vi "vipm_build.vi"   [LabVIEW 2020]
uses:
  <vilib>/Comparison/Equal/Equal Functor/Equal Functor.lvclass
  <vilib>/regexp/Match Regular Expression.xnode
  <vilib>/Wiresmith Technology/G CLI/CLI Class/CLI.lvclass
  <vilib>/Wiresmith Technology/G CLI/Argument Parser/Option Set Class/Option Set.lvclass
  <vilib>/Wiresmith Technology/G CLI/Argument Parser/Option Class/Argument Type.ctl
  <vilib>/Wiresmith Technology/G CLI/Argument Parser/Option Class/Option.lvclass
  <vilib>/Wiresmith Technology/G CLI/Argument Parser/Option Class/Option Configuration.ctl
  094f6021-4ef8-4573-82ce-a7b4949f6c5c.vi
  6795289f-0a04-455c-a499-a5e59a361415.vi
  <vilib>/Utility/error.llb/DialogType.ctl
  35111923-3b9e-4c36-b72b-79289da6bcaf.vi
  0b828e9d-cbba-40c4-b017-a79c080be190.vi
  <resource>/dialog/lvconfig.llb/LV Config Write String.vi
  <resource>/dialog/lvconfig.llb/LV Config Write Numeric (I32).vi
  <resource>/dialog/lvconfig.llb/LV Config Write Color.vi
  <resource>/dialog/lvconfig.llb/LV Config Write Pathlist.vi
  <vilib>/JKI/VIPM API/VIPM API_vipm_api.lvlib
  <resource>/dialog/lvconfig.llb/LV Config Write Boolean.vi
  0a0c95df-62a9-4167-843d-69168cea43e8.vi
  611b17c5-4e93-4ed1-8d2f-f8190cd7dade.vi
types:
  T1 = cluster{"VerboseMode":bool, "Operation":string, "Arguments":string[], "VipbFile":path}
  T2 = enum32{"Invalid", "Standard", "Closed", "Hidden", "Minimized", "Maximized"}
  T3 = typedef "Option Parser.lvlib/Option.lvclass/Option Configuration.ctl" = cluster{"Option Type":T4, "Option Labels":string[], "Key":string, "Description":string, "Required":bool, "Default Value":string}
  T4 = typedef "Option Parser.lvlib/Option.lvclass/Argument Type.ctl" = enum16{"flag", "value"}
  T5 = typedef "VIPM API_vipm_api.lvlib/VI Package Build Spec Data Cluster_vipm_api.ctl" = cluster{"Package Version":T6, "Product Name":string, "Company Name":string, "Author Name (Person or Company)":string, "Product Homepage (URL)":string, "Legal Copyright":string, "License Agreement Name":string, "Product Description Summary":string, "Product Description":string, "Release Notes - Change Log":string}
  T6 = typedef "VIPM API_vipm_api.lvlib/Version Info Cluster_vipm_api.ctl" = cluster{"major":u32, "minor":u32, "patch":u32, "build":u32}
  T7 = typedef "DialogType.ctl" = u16
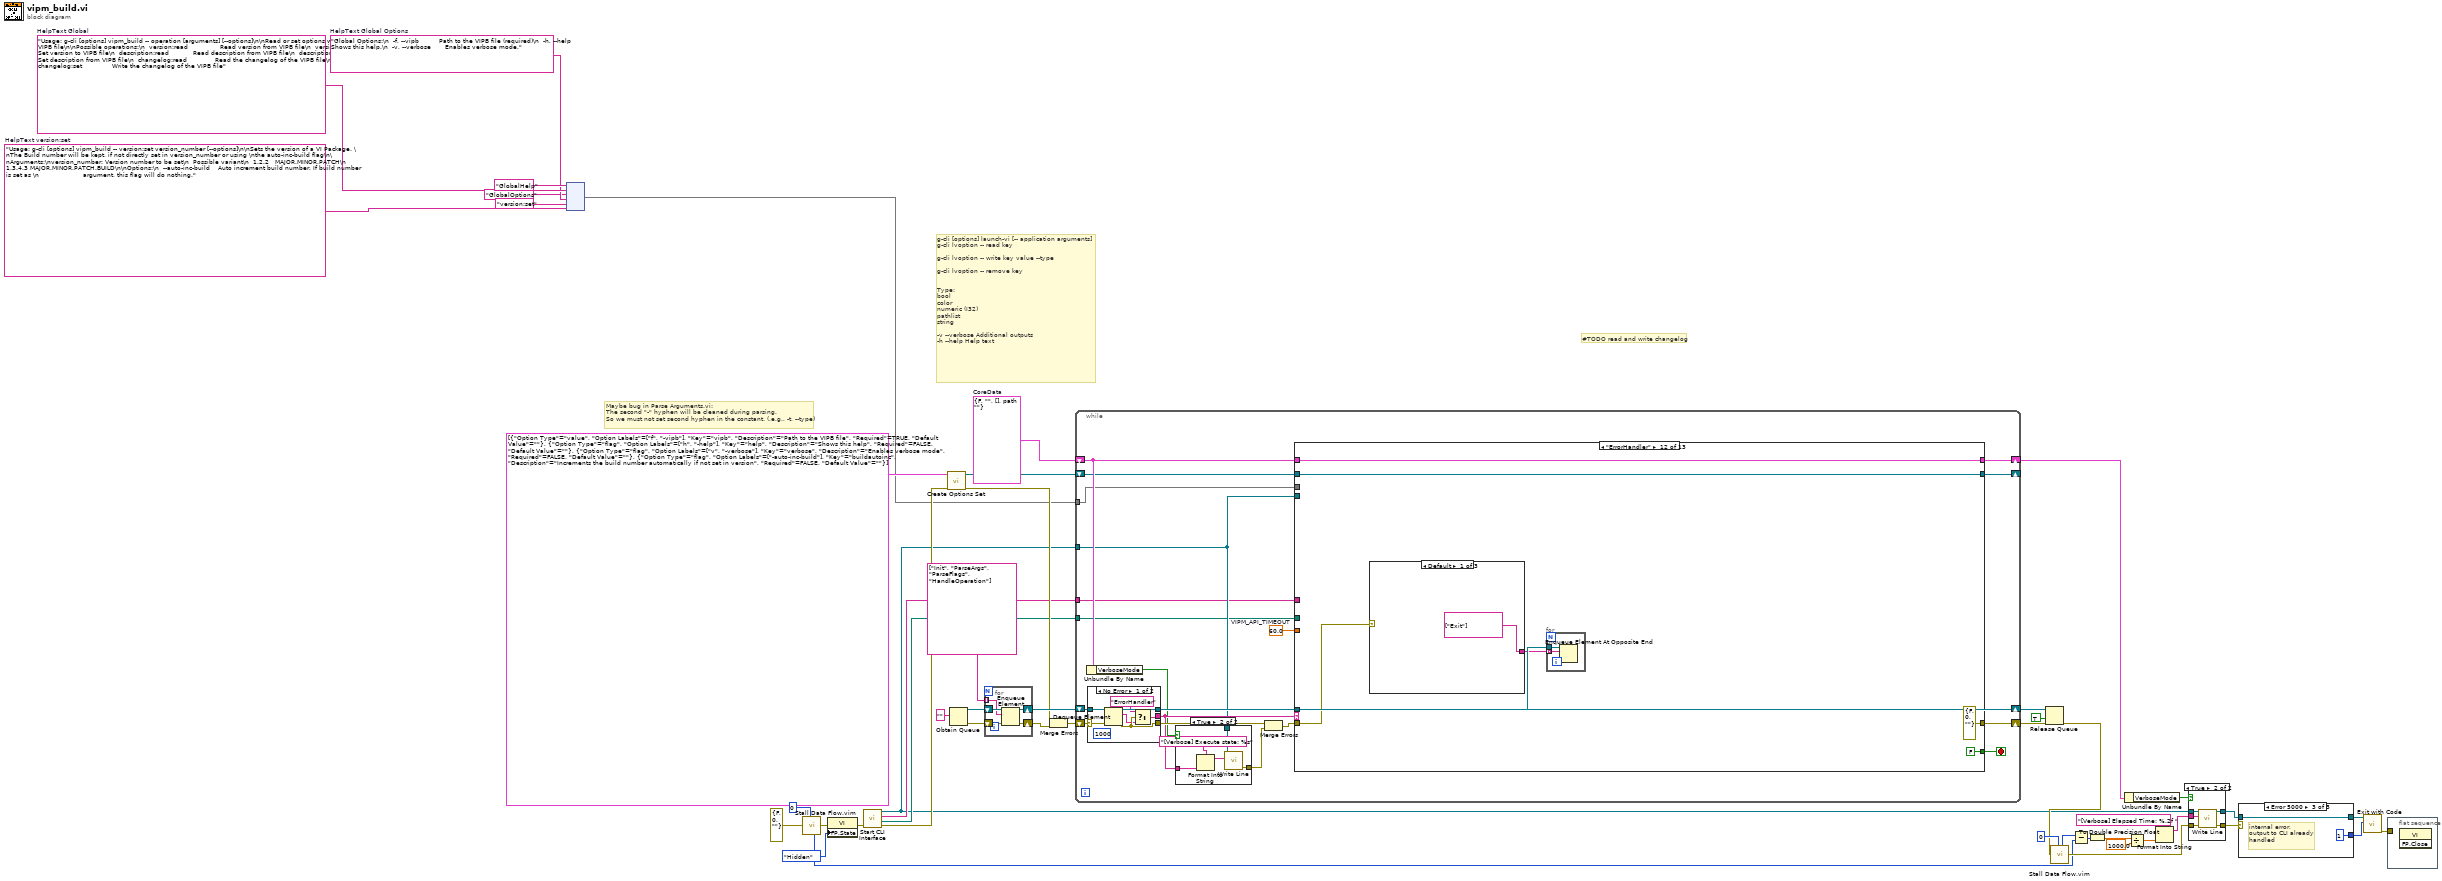
[diagram p0: block diagram]
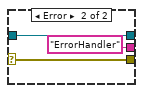
[diagram p4: hidden frame]
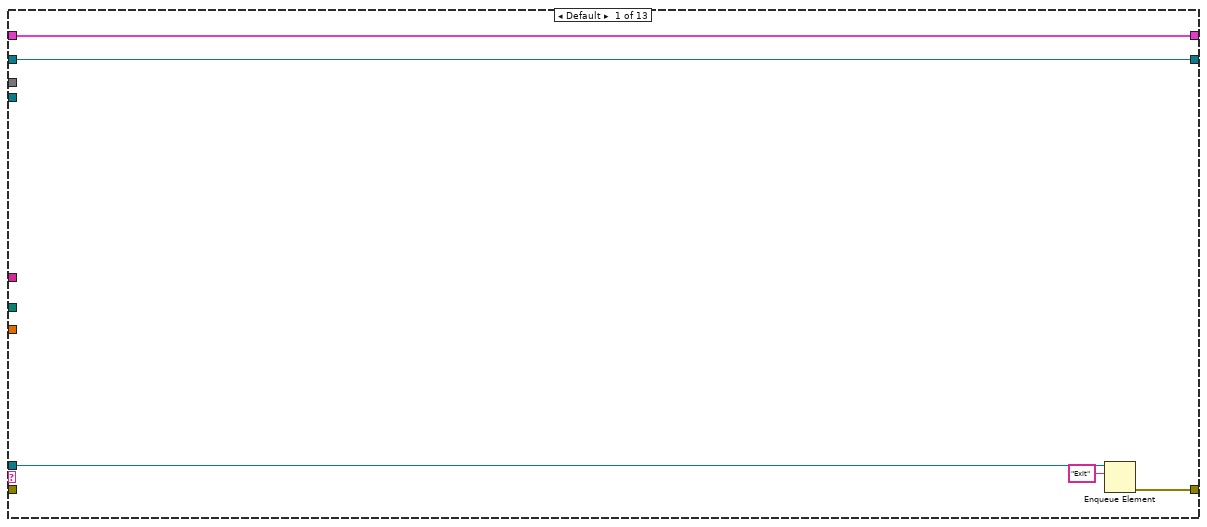
[diagram p5: hidden frame]
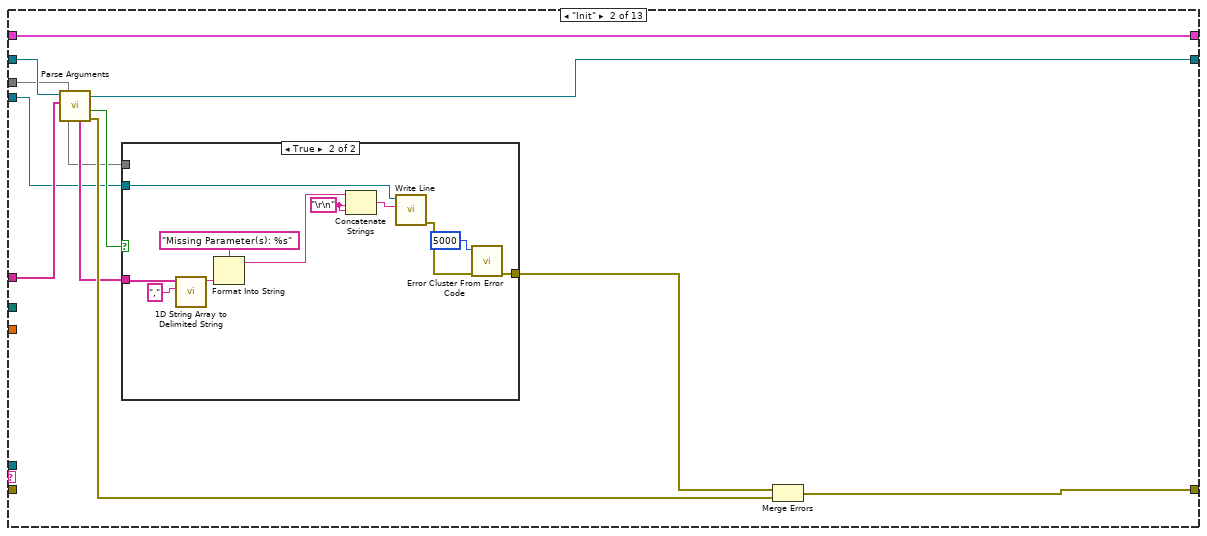
[diagram p6: hidden frame]
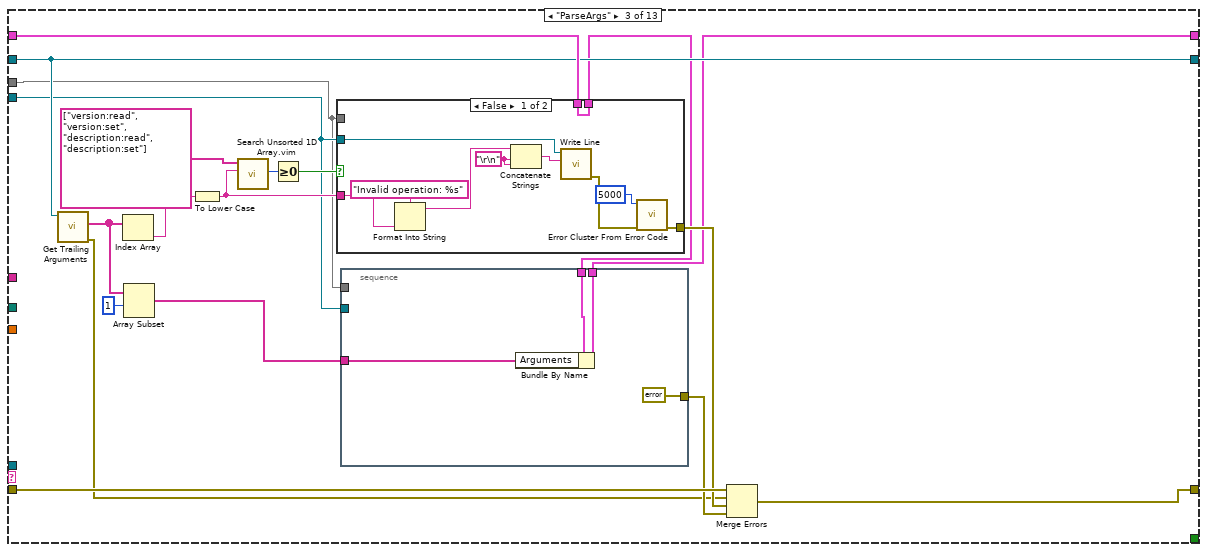
[diagram p8: hidden frame]
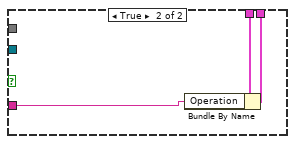
[diagram p9: hidden frame]
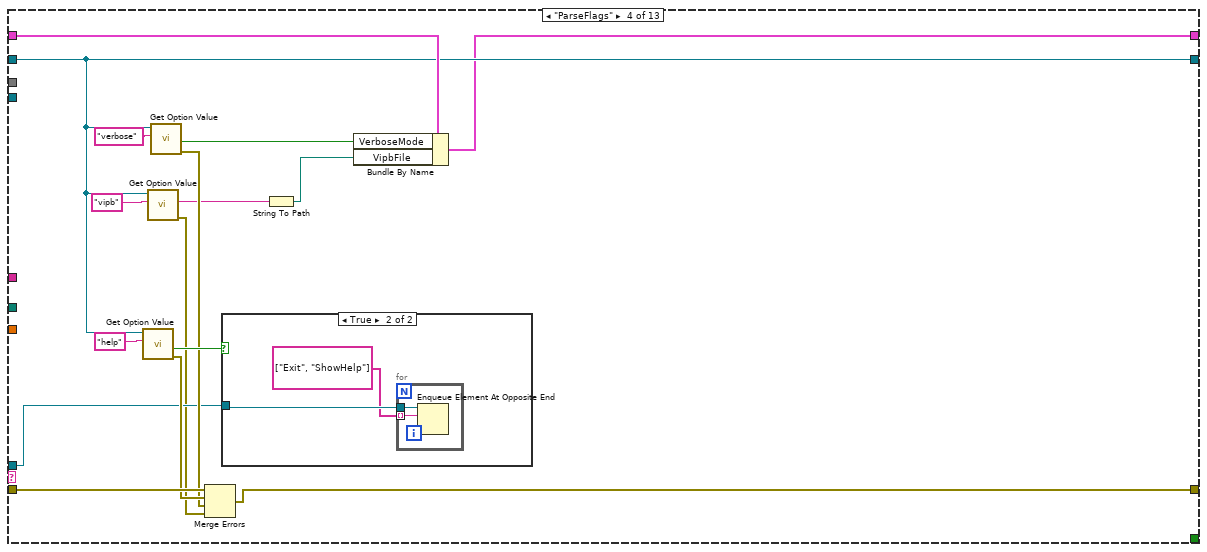
[diagram p10: hidden frame]
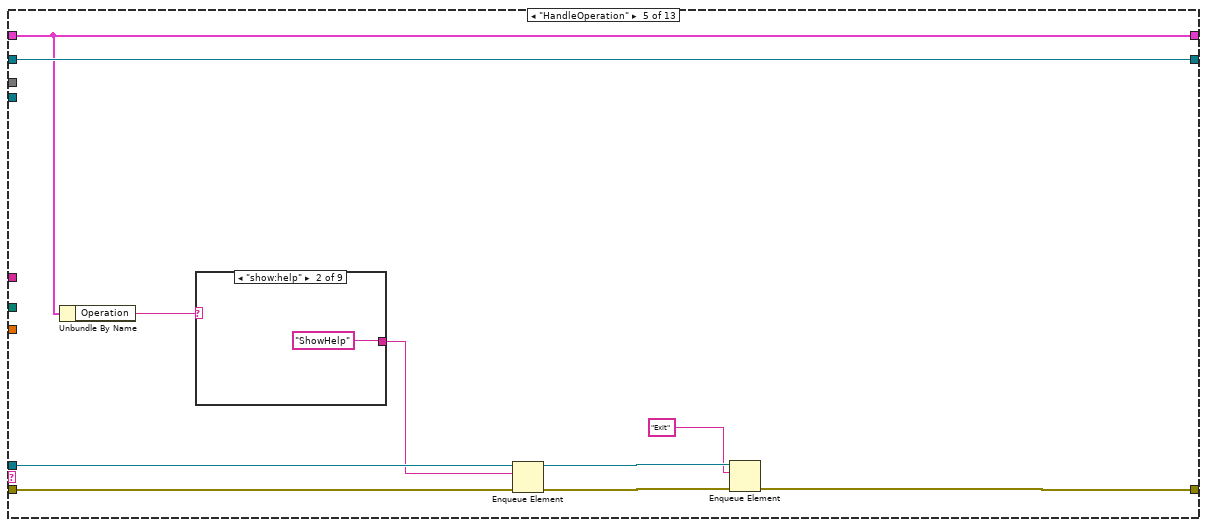
[diagram p12: hidden frame]
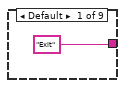
[diagram p13: hidden frame]
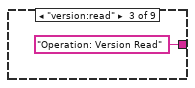
[diagram p14: hidden frame]
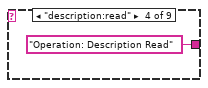
[diagram p15: hidden frame]
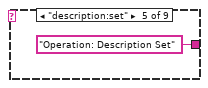
[diagram p16: hidden frame]
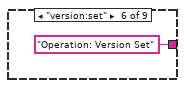
[diagram p17: hidden frame]
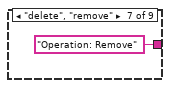
[diagram p18: hidden frame]
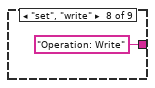
[diagram p19: hidden frame]
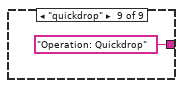
[diagram p20: hidden frame]
diagram:
  w5 = "Global Options:\n  -f, --vipb          Path to the VIPB file (required)\n  -h, --help          Shows this help.\n  -v, --verbose       Enables verbose mode."  # HelpText Global Options
  w2 = "Usage: g-cli [options] vipm_build -- version:set version_number [--options]\n\nSets the version of a VI Package. \nThe Build number will be kept, if not directly set in version_number or using \nthe auto-inc-build flag\n\nArguments:\nversion_number: Version number to be set\n  Possible variant\n  1.2.2   MAJOR.MINOR.PATCH\n  1.3.4.3 MAJOR.MINOR.PATCH.BUILD\n\nOptions:\n  --auto-inc-build    Auto increment build number. If build number is set as \n                      argument, this flag will do nothing."  # HelpText version:set
  w7 = "Usage: g-cli [options] vipm_build -- operation [arguments] [--options]\n\nRead or set options within VIPB file\n\nPossible operations:\n  version:read                Read version from VIPB file\n  version:set                 Set version to VIPB file\n  description:read            Read description from VIPB file\n  description:set             Set description from VIPB file\n  changelog:read              Read the changelog of the VIPB file\n  changelog:set               Write the changelog of the VIPB file"  # HelpText Global
  w20 = T1 {"VerboseMode"=FALSE, "Operation"="", "Arguments"=[], "VipbFile"=path ""}  # CoreData
  # "#TODO read and write changelog"
  # "Maybe bug in Parse Arguments.vi: \nThe second \"-\" hyphen will be cleaned during parsing.\nSo we must not set second hyphen in the constant. (.e.g., -t, --type)"
  # "g-cli [options] launch-vi [-- application arguments]\ng-cli lvoption -- read key\n\ng-cli lvoption -- write key value --type \n\ng-cli lvoption -- remove key\n\n\nType:\nbool\ncolor\nnumeric (I32)\npathlist\nstring\n\n-v --verbose Additional outputs\n-h --help Help text"
  n1 = node("GlobalHelp" ("key"), w7, "GlobalOptions" ("key"), w5, "version:set" ("key"), w2) -> (w1:map{string, string})
  n2 = call "Stall Data Flow.vim"("value in"=errorcluster {"status"=FALSE, "code"=0, "source"=""} ("error in (no error)"), "milliseconds to wait"=u32 0) -> ("millisecond timer value"=w36:u32, "value out"=w43:errorcluster)
  n3 = property class="VI"(error in=w43, "FP.State"=T2."Hidden" ("Front Panel Window:State")) -> (error out=w42:errorcluster)  [unwired: 1 in, 1 out]
  n4 = call <vilib>:"Start CLI Interface.vi"("error in (no error)"=w42) -> ("error out"=w47:errorcluster, "Working Directory"=w13:path, "Custom Parameters"=w14:string[], "CLI out"=w11:refnum<class "CLI.lvclass">)  [unwired: 7 in]
  n5 = call <vilib>:"Create Options Set.vi"("error in (no error)"=w47, "Options"=T3[] [{"Option Type"=enum."value", "Option Labels"=["f", "-vipb"], "Key"="vipb", "Description"="Path to the VIPB file", "Required"=TRUE, "Default Value"=""}, {"Option Type"=enum."flag", "Option Labels"=["h", "-help"], "Key"="help", "Description"="Shows this help", "Required"=FALSE, "Default Value"=""}, {"Option Type"=enum."flag", "Option Labels"=["v", "-verbose"], "Key"="verbose", "Description"="Enables verbose mode", "Required"=FALSE, "Default Value"=""}, {"Option Type"=enum."flag", "Option Labels"=["-auto-inc-build"], "Key"="buildautoinc", "Description"="Increments the build number automatically if not set in version", "Required"=FALSE, "Default Value"=""}]) -> ("error out"=w16:errorcluster, "Option Set out"=w18:refnum<class "Option Set.lvclass">)  [unwired: 8 in]
  n6 = Obtain Queue(element data type="") -> (queue out=w25:refnum<queue>, error out=w22:errorcluster)  [unwired: 4 in, 1 out]
  n7 = for {
    shift-right: [w51] -> w23
    shift-left: w25 -> [w52]
    shift-right: [w49] -> w17
    shift-left: w22 -> [w50]
    tunnel: string[] ["Init", "ParseArgs", "ParseFlags", "HandleOperation"] -> [w48] mode=indexing
    n8 = Enqueue Element(queue=w52, element=w48, error in (no error)=w50) -> (queue out=w51:refnum<queue>, error out=w49:errorcluster)  [unwired: 1 in, 1 out]
  }
  n9 = Merge Errors(w16, w17) -> (w15:errorcluster)
  n10 = while {
    shift-right: [w68] -> w10
    shift-left: w20 -> [w63]
    shift-right: [w66] -> w12
    shift-left: w15 -> [w70]
    shift-right: [w65] -> w21
    shift-left: w23 -> [w71]
    tunnel: w11 -> [w61]
    tunnel: w14 -> [w56]
    tunnel: w13 -> [w57]
    tunnel: w1 -> [w55]
    shift-right: [w54] -> _
    shift-left: w18 -> [w60]
    stop <- w67 stop-if-true
    w53 = 60.0  # VIPM_API_TIMEOUT
    n11 = Unbundle By Name(w63) -> ("VerboseMode"=w62:bool)
    n12 = case shown="No Error" w70 {
      selector: w70 -> [w82 w86]
      tunnel: w71 -> [w83 w85]
      tunnel: [w78 "ErrorHandler"] -> w64
      tunnel: [w80 w86] -> w69
      tunnel: [w81 w85] -> w65
      frame No Error {
        (unwired) 1000 ("timeout in ms (-1)")
        n13 = Dequeue Element(queue=w83, error in (no error)=w82) -> (queue out=w81:refnum<queue>, element=w79:string, error out=w80:errorcluster)  [unwired: 1 in, 1 out]
        n14 = Select(t="ErrorHandler", s=w80, f=w79) -> (s? t:f=w78:string)
      }
      frame Error {
      }
    }
    n15 = case shown="True" w62 {
      tunnel: w64 -> [_ w76]
      tunnel: w61 -> [_ w73]
      tunnel: [_ w72] -> w58
      frame False {
      }
      frame True {
        n16 = Format Into String(format string="[Verbose] Execute state: %s", w76) -> (resulting string=w74:string)  [unwired: 2 in, 1 out]
        n17 = call <vilib>:"Write Line.vi"("Text to Write"=w74, "CLI in"=w73) -> ("error out"=w72:errorcluster)  [unwired: 8 in, 1 out]
      }
    }
    n18 = Merge Errors(w69, w58) -> (w59:errorcluster)
    n19 = case shown="\"ErrorHandler\"" w64 {
      tunnel: w59 -> [_ _ w131 w162 w176 w189 w225 w264 w450 w510 _ w590 w599]
      tunnel: [w91 w102 w121 w150 w178 w207 w236 w275 w461 w507 w583 w593 w601] -> w68
      tunnel: w63 -> [w91 w102 w132 w165 w178 w207 w236 w275 w461 w507 w583 w593 w601]
      tunnel: [_ _ _ _ _ _ _ _ _ _ _ FALSE TRUE] -> w67
      tunnel: [w89 w94 w124 w160 w170 w206 w235 w274 w460 w498 w584 errorcluster {"status"=FALSE, "code"=0, "source"=""} ("error IO") w599] -> w66
      tunnel: w65 -> [w90 _ _ w156 w175 _ _ w263 w449 _ _ w589 _]
      tunnel: w61 -> [_ w95 w120 _ _ w202 w231 w258 w447 w495 w585 _ _]
      tunnel: w60 -> [w87 w101 w130 w151 w179 w208 w237 w256 w448 w505 w586 w591 w598]
      tunnel: w57 -> [_ _ _ _ _ _ _ _ _ _ _ _ _]
      tunnel: w56 -> [_ w100 _ _ _ _ _ _ _ _ _ _ _]
      tunnel: w55 -> [_ w96 w119 _ _ _ _ _ _ _ w577 _ _]
      tunnel: [w87 w92 w130 w151 w179 w208 w237 w256 w448 w505 w586 w591 w598] -> w54
      tunnel: w53 -> [_ _ _ _ _ w190 w226 w268 w454 _ _ _ _]
      frame Default {
        n20 = Enqueue Element(queue=w90, element="Exit") -> (error out=w89:errorcluster)  [unwired: 2 in, 2 out]
      }
      frame "Init" {
        n21 = call <vilib>:"Parse Arguments.vi"("Arguments"=w100, "Option Set in"=w101) -> ("error out"=w99:errorcluster, "Missing Options"=w98:bool, "Option Set out"=w92:refnum<class "Option Set.lvclass">, "Missing Option Keys"=w97:string[])  [unwired: 6 in]
        n22 = case shown="True" w98 {
          tunnel: w97 -> [_ w112]
          tunnel: w96 -> [_ _]
          tunnel: w95 -> [_ w106]
          tunnel: [_ w103] -> w93
          frame False {
          }
          frame True {
            w109 = "\r\n"
            n23 = call <vilib>:"1D String Array to Delimited String.vi"("delimiter"=",", "string array"=w112) -> ("delimited string"=w110:string)  [unwired: 9 in]
            n24 = Format Into String(format string="Missing Parameter(s): %s", w110) -> (resulting string=w108:string)  [unwired: 2 in, 1 out]
            n25 = Concatenate Strings(w108, w109, w109) -> (w107:string)
            n26 = call <vilib>:"Write Line.vi"("Text to Write"=w107, "CLI in"=w106) -> ("error out"=w104:errorcluster)  [unwired: 8 in, 1 out]
            n27 = call <vilib>:"Error Cluster From Error Code.vi"("error in (no error)"=w104, "error code (0)"=5000) -> ("error out"=w103:errorcluster)  [unwired: 7 in]
          }
        }
        n28 = Merge Errors(w93, w99) -> (w94:errorcluster)
      }
      frame "ParseArgs" {
        n29 = call <vilib>:"Get Trailing Arguments.vi"("Option Set in"=w130) -> ("error out"=w117:errorcluster, "Arguments"=w116:string[])  [unwired: 8 in, 1 out]
        n30 = Index Array(array=w116) -> (element=w129:string)  [unwired: 1 in]
        n31 = Array Subset(array=w116, index=1) -> (w114:string[])  [unwired: 1 in]
        n32 = To Lower Case(string=w129) -> (all lower case string=w125:string)
        n33 = call "Search Unsorted 1D Array.vim"("element"=w125, "unsorted 1D array"=string[] ["version:read", "version:set", "description:read", "description:set"]) -> ("index of element"=w127:i32)  [unwired: 9 in]
        n34 = Greater Or Equal To 0?(x=w127) -> (x >= 0?=w126:bool)
        n35 = case shown="False" w126 {
          tunnel: w119 -> [_ _]
          tunnel: w120 -> [w142 _]
          tunnel: [w139 _] -> w123
          tunnel: w132 -> [w137 w149]
          tunnel: w125 -> [w138 w148]
          tunnel: [w137 w147] -> w122
          frame False {
            w145 = "\r\n"
            n36 = Format Into String(format string="Invalid operation: %s", w138) -> (resulting string=w144:string)  [unwired: 2 in, 1 out]
            n37 = Concatenate Strings(w144, w145, w145) -> (w143:string)
            n38 = call <vilib>:"Write Line.vi"("Text to Write"=w143, "CLI in"=w142) -> ("error out"=w140:errorcluster)  [unwired: 8 in, 1 out]
            n39 = call <vilib>:"Error Cluster From Error Code.vi"("error in (no error)"=w140, "error code (0)"=5000) -> ("error out"=w139:errorcluster)  [unwired: 7 in]
          }
          frame True {
            n40 = Bundle By Name(cluster=w149, "Operation"=w148) -> (w147:T1)
          }
        }
        n41 = stacked-sequence {
          tunnel: w119 -> [_]
          tunnel: w120 -> [_]
          tunnel: [errorcluster {"status"=FALSE, "code"=0, "source"=""} ("error constant")] -> w118
          tunnel: w122 -> [w136]
          tunnel: w114 -> [w135]
          tunnel: [w134] -> w121
          frame #0 {
            n42 = Bundle By Name(cluster=w136, "Arguments"=w135) -> (w134:T1)
          }
        }
        n43 = Merge Errors(w131, w117, w123, w118) -> (w124:errorcluster)
      }
      frame "ParseFlags" {
        n44 = call <vilib>:"Get Option Value.vi"("Option Key"="help", "Option Set in"=w151) -> ("error out"=w159:errorcluster, "Set"=w163:bool)  [unwired: 6 in, 2 out]
        n45 = call <vilib>:"Get Option Value.vi"("Option Key"="vipb", "Option Set in"=w151) -> ("error out"=w154:errorcluster, "Value"=w152:string)  [unwired: 6 in, 2 out]
        n46 = call <vilib>:"Get Option Value.vi"("Option Key"="verbose", "Option Set in"=w151) -> ("error out"=w158:errorcluster, "Set"=w157:bool)  [unwired: 6 in, 2 out]
        n47 = Merge Errors(w162, w159, w158, w154) -> (w160:errorcluster)
        n48 = case shown="True" w163 {
          tunnel: w156 -> [_ w167]
          frame False {
          }
          frame True {
            n49 = for {
              tunnel: w167 -> [w169]
              tunnel: string[] ["Exit", "ShowHelp"] -> [w168] mode=indexing
              n50 = Enqueue Element At Opposite End(queue=w169, element=w168) -> ()  [unwired: 2 in, 3 out]
            }
          }
        }
        n51 = String To Path(string=w152) -> (path=w153:path)
        n52 = Bundle By Name(cluster=w165, "VerboseMode"=w157, "VipbFile"=w153) -> (w150:T1)
      }
      frame "HandleOperation" {
        n53 = Unbundle By Name(w178) -> ("Operation"=w177:string)
        n54 = case shown="\"show:help\"" w177 {
          tunnel: ["Exit" "ShowHelp" "Operation: Version Read" "Operation: Description Read" "Operation: Description Set" "Operation: Version Set" "Operation: Remove" "Operation: Write" "Operation: Quickdrop"] -> w174
          frame Default {
          }
          frame "show:help" {
          }
          frame "version:read" {
          }
          frame "description:read" {
          }
          frame "description:set" {
          }
          frame "version:set" {
          }
          frame "delete", "remove" {
          }
          frame "set", "write" {
          }
          frame "quickdrop" {
          }
        }
        n55 = Enqueue Element(queue=w175, element=w174, error in (no error)=w176) -> (queue out=w172:refnum<queue>, error out=w173:errorcluster)  [unwired: 1 in, 1 out]
        n56 = Enqueue Element(queue=w172, element="Exit", error in (no error)=w173) -> (error out=w170:errorcluster)  [unwired: 1 in, 2 out]
      }
      frame "Operation: Version Read" {
        n57 = Unbundle By Name(w207) -> ("VerboseMode"=w203:bool, "VipbFile"=w201:path)
        n58 = case shown="True" w203 {
          tunnel: w202 -> [_ w211]
          tunnel: [_ w210] -> w199
          frame False {
          }
          frame True {
            n59 = call <vilib>:"Write Line.vi"("Text to Write"="[Verbose] Read version" ("format string"), "CLI in"=w211) -> ("error out"=w210:errorcluster)  [unwired: 8 in, 1 out]
          }
        }
        n60 = call <vilib>:"Read VI Package Build Spec_vipm_api.vi"("Timeout in seconds (0: no timeout)"=w190, "error in (no error)"=w199, "Path to VIPB File"=w201) -> ("error out"=w198:errorcluster, "VI Package Build Spec Data"=w200:T5)  [unwired: 7 in]
        n61 = Unbundle By Name(w200) -> ("Package Version"=w197:T6)
        n62 = Unbundle(w197) -> ("major"=w196:u32, "minor"=w195:u32, "patch"=w194:u32, "build"=w193:u32)
        n63 = Format Into String(format string="%d.%d.%d.%d", w196, w195, w194, w193) -> (resulting string=w192:string)  [unwired: 2 in, 1 out]
        n64 = case shown="No Error" w198 {
          selector: w198 -> [_ w218]
          tunnel: [w213 w221] -> w204
          tunnel: w202 -> [w214 w220]
          tunnel: w192 -> [w212 _]
          frame No Error {
            n65 = call <vilib>:"Write Line.vi"("Text to Write"=w212, "CLI in"=w214) -> ("error out"=w213:errorcluster)  [unwired: 8 in, 1 out]
          }
          frame Error {
            w219 = T7 0 items=["no dialog", "OK message", "continue or stop message", "OK message + warnings", "continue/stop + warnings"] ("type of dialog (OK msg:1)")
            n66 = call <vilib>:"Simple Error Handler.vi"("type of dialog (OK msg:1)"=w219, "error in (no error)"=w218) -> ("message"=w215:string)  [unwired: 3 in, 4 out]
            n67 = Format Into String(format string="Error: '%s'", w215) -> (resulting string=w217:string)  [unwired: 2 in, 1 out]
            n68 = call <vilib>:"Write Line.vi"("Text to Write"=w217, "CLI in"=w220) -> ("error out"=w222:errorcluster)  [unwired: 8 in, 1 out]
            n69 = call <vilib>:"Error Cluster From Error Code.vi"("error in (no error)"=w222, "error code (0)"=5000) -> ("error out"=w221:errorcluster)  [unwired: 7 in]
          }
        }
        n70 = Merge Errors(w204, w198) -> (w205:errorcluster)
        n71 = Merge Errors(w189, w205) -> (w206:errorcluster)
      }
      frame "Operation: Description Read" {
        # "#TODO read description to file"
        n72 = Unbundle By Name(w236) -> ("VerboseMode"=w232:bool, "VipbFile"=w230:path)
        n73 = case shown="True" w232 {
          tunnel: w231 -> [_ w240]
          tunnel: [_ w239] -> w228
          frame False {
          }
          frame True {
            n74 = call <vilib>:"Write Line.vi"("Text to Write"="[Verbose] Read description" ("format string"), "CLI in"=w240) -> ("error out"=w239:errorcluster)  [unwired: 8 in, 1 out]
          }
        }
        n75 = call <vilib>:"Read VI Package Build Spec_vipm_api.vi"("Timeout in seconds (0: no timeout)"=w226, "error in (no error)"=w228, "Path to VIPB File"=w230) -> ("error out"=w227:errorcluster, "VI Package Build Spec Data"=w229:T5)  [unwired: 7 in]
        n76 = Unbundle By Name(w229) -> ("Product Description"=w224:string)
        n77 = case shown="No Error" w227 {
          selector: w227 -> [_ w247]
          tunnel: [w242 w250] -> w233
          tunnel: w231 -> [w243 w249]
          tunnel: w224 -> [w241 _]
          frame No Error {
            n78 = call <vilib>:"Write Line.vi"("Text to Write"=w241, "CLI in"=w243) -> ("error out"=w242:errorcluster)  [unwired: 8 in, 1 out]
          }
          frame Error {
            w248 = T7 0 items=["no dialog", "OK message", "continue or stop message", "OK message + warnings", "continue/stop + warnings"] ("type of dialog (OK msg:1)")
            n79 = call <vilib>:"Simple Error Handler.vi"("type of dialog (OK msg:1)"=w248, "error in (no error)"=w247) -> ("message"=w244:string)  [unwired: 3 in, 4 out]
            n80 = Format Into String(format string="Error: '%s'", w244) -> (resulting string=w246:string)  [unwired: 2 in, 1 out]
            n81 = call <vilib>:"Write Line.vi"("Text to Write"=w246, "CLI in"=w249) -> ("error out"=w251:errorcluster)  [unwired: 8 in, 1 out]
            n82 = call <vilib>:"Error Cluster From Error Code.vi"("error in (no error)"=w251, "error code (0)"=5000) -> ("error out"=w250:errorcluster)  [unwired: 7 in]
          }
        }
        n83 = Merge Errors(w233, w227) -> (w234:errorcluster)
        n84 = Merge Errors(w225, w234) -> (w235:errorcluster)
      }
      frame "Operation: Version Set" {
        n85 = Unbundle By Name(w275) -> ("VerboseMode"=w273:bool, "VipbFile"=w266:path, "Arguments"=w271:string[])
        n86 = Index Array(array=w271) -> (element=w259:string)  [unwired: 1 in]
        n87 = case shown="True" w273 {
          tunnel: w258 -> [_ w444]
          tunnel: [_ w443] -> w272
          frame False {
          }
          frame True {
            n88 = call <vilib>:"Write Line.vi"("Text to Write"="[Verbose] Set version" ("format string"), "CLI in"=w444) -> ("error out"=w443:errorcluster)  [unwired: 8 in, 1 out]
          }
        }
        n89 = call <vilib>:"Get Option Value.vi"("Option Key"="buildautoinc", "Option Set in"=w256) -> ("error out"=w254:errorcluster, "Set"=w253:bool)  [unwired: 6 in, 2 out]
        n90 = call <vilib>:"Read VI Package Build Spec_vipm_api.vi"("Timeout in seconds (0: no timeout)"=w268, "error in (no error)"=w272, "Path to VIPB File"=w266) -> ("error out"=w270:errorcluster, "VI Package Build Spec Data"=w267:T5)  [unwired: 7 in]
        n91 = xnode "Match Regular Expression"("input string"=w259, "regular expression"="^v?\\d+.\\d+.\\d+(?:.\\d+)?$") -> ("offset past match"=w261:i32)  [unwired: 4 in, 4 out]
        n92 = Greater Or Equal To 0?(x=w261) -> (x >= 0?=w260:bool)
        n93 = Merge Errors(w264, w254) -> (w255:errorcluster)
        n94 = case shown="True" w260 {
          tunnel: [w283 w290] -> w269
          tunnel: w268 -> [_ w309]
          tunnel: w267 -> [_ w308]
          tunnel: w266 -> [_ w307]
          tunnel: w270 -> [_ w303]
          tunnel: w259 -> [w282 w298]
          tunnel: w258 -> [w281 _]
          tunnel: w253 -> [_ w288]
          frame False {
            n95 = Format Into String(format string="Invalid version argument: '%s' (expected format: [v]0.3.2.4)", w282) -> (resulting string=w285:string)  [unwired: 2 in, 1 out]
            n96 = call <vilib>:"Write Line.vi"("Text to Write"=w285, "CLI in"=w281) -> ("error out"=w286:errorcluster)  [unwired: 8 in, 1 out]
            n97 = call <vilib>:"Error Cluster From Error Code.vi"("error in (no error)"=w286, "error code (0)"=5000) -> ("error out"=w283:errorcluster)  [unwired: 7 in]
          }
          frame True {
            n98 = Search and Replace String(input string=w298, search string="^v") -> (result string=w301:string, error out=w299:errorcluster)  [unwired: 6 in, 2 out]
            n99 = Merge Errors(w303, w299) -> (w300:errorcluster)
            n100 = call <vilib>:"Delimited String to 1D String Array.vi"("delimiter"=".", "delimited string"=w301) -> ("string array"=w312:string[])  [unwired: 9 in]
            n101 = Decimal String To Number(string=w312, default (0L)=u32 0 ("default (0 I32)")) -> (number=w297:u32[])  [unwired: 1 in, 1 out]
            n102 = Array Size(array=w297) -> (size(s)=w296:i32)
            n103 = Index Array(array=w297) -> (element #1=w306:u32, element #2=w305:u32, element #3=w304:u32, element #4=w292:u32)  [unwired: 4 in]
            n104 = Greater Or Equal?(x=w296, y=4) -> (x >= y?=w291:bool)
            n105 = Bundle By Name(cluster=w308, "Package Version.major"=w306, "Package Version.minor"=w305, "Package Version.patch"=w304) -> (w294:T5)
            n106 = case shown="False" w291 {
              tunnel: w294 -> [w315 w324]
              tunnel: [w316 w323] -> w293
              tunnel: w292 -> [_ w322]
              tunnel: w288 -> [w314 _]
              frame False {
                n107 = case shown="True" w314 {
                  tunnel: [w317 w321] -> w316
                  tunnel: w315 -> [w317 w320]
                  frame False {
                  }
                  frame True {
                    # "Auto inc build number if set"
                    n108 = Unbundle By Name(w320) -> ("Package Version.build"=w318:u32)
                    n109 = Increment(x=w318) -> (x+1=w319:u32)
                    n110 = Bundle By Name(cluster=w320, "Package Version.build"=w319) -> (w321:T5)
                  }
                }
              }
              frame True {
                # "Set the build number from argument"
                n111 = Bundle By Name(cluster=w324, "Package Version.build"=w322) -> (w323:T5)
              }
            }
            n112 = call <vilib>:"Write VI Package Build Spec_vipm_api.vi"("Timeout in seconds (0: no timeout)"=w309, "error in (no error)"=w300, "VI Package Build Spec Data"=w293, "Path to VIPB File"=w307) -> ("error out"=w310:errorcluster)  [unwired: 7 in]
            n113 = call "Stall Data Flow.vim"("value in"=w310, "milliseconds to wait"=u32 500) -> ("value out"=w290:errorcluster)  [unwired: 1 out]
          }
        }
        n114 = disable-structure shown="Enabled" {
          disable-tunnel: [w278 w280] -> w265
          disable-tunnel: w255 -> [w277 w280]
          disable-tunnel: w263 -> [w276 _]
          frame Disabled {
            n115 = Enqueue Element At Opposite End(queue=w276, element="Operation: Version Read", error in (no error)=w277) -> (error out=w278:errorcluster)  [unwired: 1 in, 2 out]
          }
          frame Enabled {
          }
        }
        n116 = Merge Errors(w265, w269) -> (w274:errorcluster)
      }
      frame "Operation: Description Set" {
        n117 = Unbundle By Name(w461) -> ("VerboseMode"=w459:bool, "VipbFile"=w452:path, "Arguments"=w457:string[])
        n118 = Index Array(array=w457) -> (element=w445:string)  [unwired: 1 in]
        n119 = case shown="True" w459 {
          tunnel: w447 -> [_ w485]
          tunnel: [_ w484] -> w458
          frame False {
          }
          frame True {
            n120 = call <vilib>:"Write Line.vi"("Text to Write"="[Verbose] Set description" ("format string"), "CLI in"=w485) -> ("error out"=w484:errorcluster)  [unwired: 8 in, 1 out]
          }
        }
        n121 = call <vilib>:"Read VI Package Build Spec_vipm_api.vi"("Timeout in seconds (0: no timeout)"=w454, "error in (no error)"=w458, "Path to VIPB File"=w452) -> ("error out"=w456:errorcluster, "VI Package Build Spec Data"=w453:T5)  [unwired: 7 in]
        n122 = Empty String/Path?(string/path=w445) -> (empty?=w446:bool)
        n123 = case shown="False" w446 {
          tunnel: [w469 w476] -> w455
          tunnel: w454 -> [_ w481]
          tunnel: w453 -> [_ w480]
          tunnel: w452 -> [_ w479]
          tunnel: w456 -> [_ w478]
          tunnel: w445 -> [_ w472]
          tunnel: w447 -> [w468 _]
          frame True {
            n124 = call <vilib>:"Write Line.vi"("Text to Write"="Empty description argument" ("format string"), "CLI in"=w468) -> ("error out"=w470:errorcluster)  [unwired: 8 in, 1 out]
            n125 = call <vilib>:"Error Cluster From Error Code.vi"("error in (no error)"=w470, "error code (0)"=5000) -> ("error out"=w469:errorcluster)  [unwired: 7 in]
          }
          frame False {
            # "#TODO read description from given file"
            n126 = String To Path(string=w472) -> (path=w474:path)
            n127 = Read from Text File(file (use dialog)=w474) -> (text=w473:string)  [unwired: 3 in, 3 out]
            n128 = Bundle By Name(cluster=w480, "Product Description"=w473) -> (w477:T5)
            n129 = call <vilib>:"Write VI Package Build Spec_vipm_api.vi"("Timeout in seconds (0: no timeout)"=w481, "error in (no error)"=w478, "VI Package Build Spec Data"=w477, "Path to VIPB File"=w479) -> ("error out"=w482:errorcluster)  [unwired: 7 in]
            n130 = call "Stall Data Flow.vim"("value in"=w482, "milliseconds to wait"=u32 500) -> ("value out"=w476:errorcluster)  [unwired: 1 out]
          }
        }
        n131 = disable-structure shown="Enabled" {
          disable-tunnel: [w464 w466] -> w451
          disable-tunnel: w450 -> [w463 w466]
          disable-tunnel: w449 -> [w462 _]
          frame Disabled {
            n132 = Enqueue Element At Opposite End(queue=w462, element="Operation: Version Read", error in (no error)=w463) -> (error out=w464:errorcluster)  [unwired: 1 in, 2 out]
          }
          frame Enabled {
          }
        }
        n133 = Merge Errors(w451, w455) -> (w460:errorcluster)
      }
      frame "Operation: Write" {
        w489 = string[] ["bool", "color", "int", "pathlist", "string"]
        # "value"
        n134 = Unbundle By Name(w507) -> ("VerboseMode"=w506:bool, "Arguments"=w487:string[])
        n135 = call <vilib>:"Get Trailing Arguments.vi"("Option Set in"=w505) -> ("error out"=w501:errorcluster, "Arguments"=w499:string[])  [unwired: 8 in, 1 out]
        n136 = call <vilib>:"Get Option Value.vi"("Option Key"="datatype", "Option Set in"=w505) -> ("error out"=w500:errorcluster, "Set"=w508:bool, "Value"=w492:string)  [unwired: 6 in, 1 out]
        n137 = Merge Errors(w510, w500, w501) -> (w502:errorcluster)
        n138 = Array Size(array=w499) -> (size(s)=w504:i32)
        n139 = call "Search Unsorted 1D Array.vim"("element"=w492, "unsorted 1D array"=w489) -> ("index of element"=w493:i32)  [unwired: 9 in]
        n140 = Index Array(array=w499, index=2) -> (element=w486:string)
        n141 = case shown="True" w506 {
          tunnel: w492 -> [_ w573]
          tunnel: w508 -> [_ w572]
          tunnel: w495 -> [w563 w569]
          tunnel: [w563 w568] -> w496
          tunnel: [_ w567] -> _
          tunnel: w487 -> [_ w566]
          tunnel: w486 -> [_ w565]
          frame False {
          }
          frame True {
            n142 = Index Array(array=w566) -> (element=w564:string)  [unwired: 1 in]
            n143 = Format Into String(format string="[Verbose] Write key'%s' with value '%s' (Datatype: '%s' CLI set: %s)", w564, w565, w573, w572) -> (resulting string=w570:string)  [unwired: 2 in, 1 out]
            n144 = call <vilib>:"Write Line.vi"("Text to Write"=w570, "CLI in"=w569) -> ("error out"=w567:errorcluster, "CLI out"=w568:refnum<class "CLI.lvclass">)  [unwired: 8 in]
          }
        }
        n145 = Greater Or Equal To 0?(x=w493) -> (x >= 0?=w491:bool)
        n146 = Greater Or Equal?(x=w504, y=3) -> (x >= y?=w490:bool)
        n147 = Compound Arithmetic op=AND(w490, w491) -> (w494:bool)
        n148 = case shown="True" w494 {
          tunnel: w496 -> [w515 w528]
          tunnel: [w514 w529] -> w497
          tunnel: w492 -> [w512 w530]
          tunnel: w491 -> [w513 _]
          tunnel: w489 -> [w511 _]
          tunnel: w487 -> [_ w531]
          tunnel: w486 -> [_ w527]
          frame False {
            n149 = case shown="False" w513 {
              tunnel: ["Value argument not provided for write operation" ("format string") w525] -> w516
              tunnel: w512 -> [_ w523]
              tunnel: w511 -> [_ w522]
              frame True {
              }
              frame False {
                n150 = call <vilib>:"1D String Array to Delimited String.vi"("delimiter"=",", "string array"=w522) -> ("delimited string"=w520:string)  [unwired: 9 in]
                n151 = Format Into String(format string="Datatype '%s' not allowed. Possible values [%s]", w523, w520) -> (resulting string=w525:string)  [unwired: 2 in, 1 out]
              }
            }
            n152 = call <vilib>:"Write Line.vi"("Text to Write"=w516, "CLI in"=w515) -> ("error out"=w517:errorcluster)  [unwired: 8 in, 1 out]
            n153 = call <vilib>:"Error Cluster From Error Code.vi"("error in (no error)"=w517, "error code (0)"=5000) -> ("error out"=w514:errorcluster)  [unwired: 7 in]
          }
          frame True {
            n154 = Index Array(array=w531) -> (element=w526:string)  [unwired: 1 in]
            n155 = case shown="\"color\"" w530 {
              tunnel: w526 -> [w533 w537 w543 w546 w557]
              tunnel: [w534 w538 w542 w545 w556] -> w529
              tunnel: w528 -> [_ _ _ w544 _]
              tunnel: w527 -> [w532 w535 w541 _ w555]
              frame "string", Default {
                n156 = call-poly <resource>:"LV Config Write.vi"("value"=w532, "key"=w533) -> ("error out"=w534:errorcluster)  [unwired: 5 in]
              }
              frame "bool" {
                n157 = case shown="\"0\", \"disable\", \"disabled\", \"False\", \"off\", Default" w535 {
                  tunnel: [_ TRUE] -> w536
                  frame "0", "disable", "disabled", "False", "off", Default {
                  }
                  frame "1", "enable", "enabled", "on", "True" {
                  }
                }
                n158 = call-poly <resource>:"LV Config Write.vi"("value"=w536, "key"=w537) -> ("error out"=w538:errorcluster)  [unwired: 5 in]
              }
              frame "int" {
                n159 = Decimal String To Number(string=w541) -> (number=w540:i32)  [unwired: 2 in, 1 out]
                n160 = call-poly <resource>:"LV Config Write.vi"("value"=w540, "key"=w543) -> ("error out"=w542:errorcluster)  [unwired: 5 in]
              }
              frame "color" {
                n161 = disable-structure shown="Disabled" {
                  disable-tunnel: w546 -> [w549 _]
                  disable-tunnel: [w548 w551] -> w545
                  disable-tunnel: w544 -> [_ w550]
                  frame Disabled {
                    # "#TODO scan from hex (HTML) or RGB\nHex: #F54927\nRGB: 245, 73, 39"
                    n162 = call <vilib>:"RGB to Color.vi"() -> ("Color"=w547:u32)  [unwired: 3 in]
                    n163 = call-poly <resource>:"LV Config Write.vi"("value"=w547, "key"=w549) -> ("error out"=w548:errorcluster)  [unwired: 5 in]
                  }
                  frame Enabled {
                    n164 = call <vilib>:"Write Line.vi"("Text to Write"="Operation 'Write' for datatype 'color' not implemented" ("format string"), "CLI in"=w550) -> ("error out"=w553:errorcluster)  [unwired: 8 in, 1 out]
                    n165 = call <vilib>:"Error Cluster From Error Code.vi"("error in (no error)"=w553, "error code (0)"=5000) -> ("error out"=w551:errorcluster)  [unwired: 7 in]
                  }
                }
              }
              frame "pathlist" {
                n166 = disable-structure shown="Enabled" {
                  disable-tunnel: w557 -> [w559 w561]
                  disable-tunnel: [w558 w560] -> w556
                  disable-tunnel: w555 -> [_ w562]
                  frame Disabled {
                    n167 = call-poly <resource>:"LV Config Write.vi"("key"=w559) -> ("error out"=w558:errorcluster)  [unwired: 6 in]
                  }
                  frame Enabled {
                    # "do not convert value: list must be separated by ';' semi-colon"
                    n168 = call-poly <resource>:"LV Config Write.vi"("value"=w562, "key"=w561) -> ("error out"=w560:errorcluster)  [unwired: 5 in]
                  }
                }
              }
            }
          }
        }
        n169 = Merge Errors(w502, w497) -> (w498:errorcluster)
      }
      frame "ShowHelp" {
        w580 = "\r\n"
        # "Use global help as default"
        n170 = Unbundle By Name(w583) -> ("Operation"=w576:string)
        n171 = Look In Map(map=w577, key="GlobalOptions") -> (value=w581:string)  [unwired: 1 in, 1 out]
        n172 = Look In Map(map=w577, key="GlobalHelp") -> (value=w575:string)  [unwired: 1 in, 1 out]
        n173 = Look In Map(map=w577, key=w576, default value=w575) -> (value=w574:string)  [unwired: 1 out]
        n174 = Concatenate Strings(w574, w580, w580, w581) -> (w579:string)
        n175 = call <vilib>:"Write Line.vi"("Text to Write"=w579, "CLI in"=w585) -> ("error out"=w584:errorcluster)  [unwired: 8 in, 1 out]
      }
      frame "ErrorHandler" {
        n176 = case shown="Default" w590 {
          tunnel: [string[] ["Exit"] _ string[] ["Exit", "ShowHelp"]] -> w588
          frame Default {
          }
          frame No Error {
          }
          frame Error {
          }
        }
        n177 = for {
          tunnel: w589 -> [w595]
          tunnel: w588 -> [w594] mode=indexing
          n178 = Enqueue Element At Opposite End(queue=w595, element=w594) -> ()  [unwired: 2 in, 3 out]
        }
      }
      frame "Exit" {
      }
    }
  }
  n179 = Release Queue(queue=w21, force destroy? (F)=TRUE) -> ()  [unwired: 1 in, 3 out]
  n180 = call "Stall Data Flow.vim"("value in"=w12, "milliseconds to wait"=u32 0) -> ("millisecond timer value"=w37:u32, "value out"=w45:errorcluster)
  n181 = Subtract(x=w37, y=w36) -> (x-y=w35:u32)
  n182 = To Double Precision Float(number=w35) -> (double precision float=w34:dbl)
  n183 = Unbundle By Name(w10) -> ("VerboseMode"=w9:bool)
  n184 = Divide(x=w34, y=1000.0) -> (x/y=w32:dbl)
  n185 = Format Into String(format string="[Verbose] Elapsed Time: %.2f ", w32) -> (resulting string=w30:string)  [unwired: 2 in, 1 out]
  n186 = case shown="True" w9 {
    tunnel: w45 -> [w602 w608]
    tunnel: [w602 w607] -> w44
    tunnel: w11 -> [w603 w606]
    tunnel: w30 -> [_ w605]
    tunnel: [w603 w604] -> w29
    frame False {
    }
    frame True {
      n187 = call <vilib>:"Write Line.vi"("error in (no error)"=w608, "Text to Write"=w605, "CLI in"=w606) -> ("error out"=w607:errorcluster, "CLI out"=w604:refnum<class "CLI.lvclass">)  [unwired: 7 in]
    }
  }
  n188 = case shown="Error 5000" w44 {
    selector: w44 -> [_ w615 _]
    tunnel: w29 -> [w609 w614 w616]
    tunnel: [w609 w613 w616] -> w28
    tunnel: [_ w610 1 ("code out")] -> w27
    frame No Error {
    }
    frame Default {
      w612 = T7 0 items=["no dialog", "OK message", "continue or stop message", "OK message + warnings", "continue/stop + warnings"] ("type of dialog (OK msg:1)")
      n189 = call <vilib>:"Simple Error Handler.vi"("type of dialog (OK msg:1)"=w612, "error in (no error)"=w615) -> ("code out"=w610:i32, "message"=w611:string)  [unwired: 3 in, 3 out]
      n190 = call <vilib>:"Write Line.vi"("Text to Write"=w611, "CLI in"=w614) -> ("CLI out"=w613:refnum<class "CLI.lvclass">)  [unwired: 8 in, 1 out]
    }
    frame Error {
      # "internal error, \noutput to CLI already\nhandled"
    }
  }
  n191 = call <vilib>:"Exit with Code.vi"("Exit Code (0)"=w27, "CLI in"=w28) -> ("error out"=w41:errorcluster)  [unwired: 9 in]
  n192 = flat-sequence {
    tunnel: w41 -> [_]
    frame #0 {
      n193 = invoke class="VI" method="FP.Close"() -> ()  [unwired: 3 in, 3 out]
    }
  }
